vi "Omniax_mDrive_COM9_MM_BR_RES.vi"() -> ()   [LabVIEW 2009]
uses:
  <vilib>/Instr/_visa.llb/VISA Configure Serial Port (Instr).vi
panel:
  out "Y Backlash corr":bool
  in  "Y Scan set":bool
  in  "Y Scan Velocity SP mm/sec":dbl
  in  "Y Scan Length SP mm":dbl
  in  "Y Move Set":bool
  out "Y Backlash steps/sec":i32
  out "Y Backlash":i32
  out "Y in Motion":bool
  in  "Reset":bool
  out "Reset Y Motor Steps":i32
  in  "Reset Y Position mm":dbl
  out "Y Velocity MV mm/sec":dbl
  in  "Y Velocity SP mm/sec":dbl
  in  "Y Position SP mm":dbl
  out "Y Position MV mm":dbl
  out "Y Holding Current %":i32
  out "Y Run Current %":i32
  out "Y Scan velocity MV mm/sec":dbl format="%#_6f"
  out "Y Scan length MV mm":dbl
  in  "Y Scan Cancel":bool
  out "Y Position mm PV":dbl
  out "Y offset mm":dbl
  out "Y mm/rev":dbl
  out "Y steps/rev":u32
  out "Y scan steps/sec MV step/sec":i32
  in  "Y Scan Length SP steps":i32 min=-460800 max=460800 step=100
  out "Y Scan":bool
  in  "Y Scan Set":bool
  in  "Scan Go":bool
  in  "Y Velocity SP step/sec":i32 min=1 max=102400
  in  "Y Scan Velocity SP steps/sec":i32=1 min=1 max=102400 step=1
  in  "Stop":bool
  out "Y in Range":bool
  out "Y Step PV":i32 max=2000
  in  "Go":bool
  in  "Y Step SP":i32=-20000 min=-460800 max=460800 step=500
  out "Y MINPOS":i32=-94296
  out "Y MAXPOS":i32=-34296
  out "Y COM PORT":refnum<visa-resource-name>="COM5"
  # "MY"
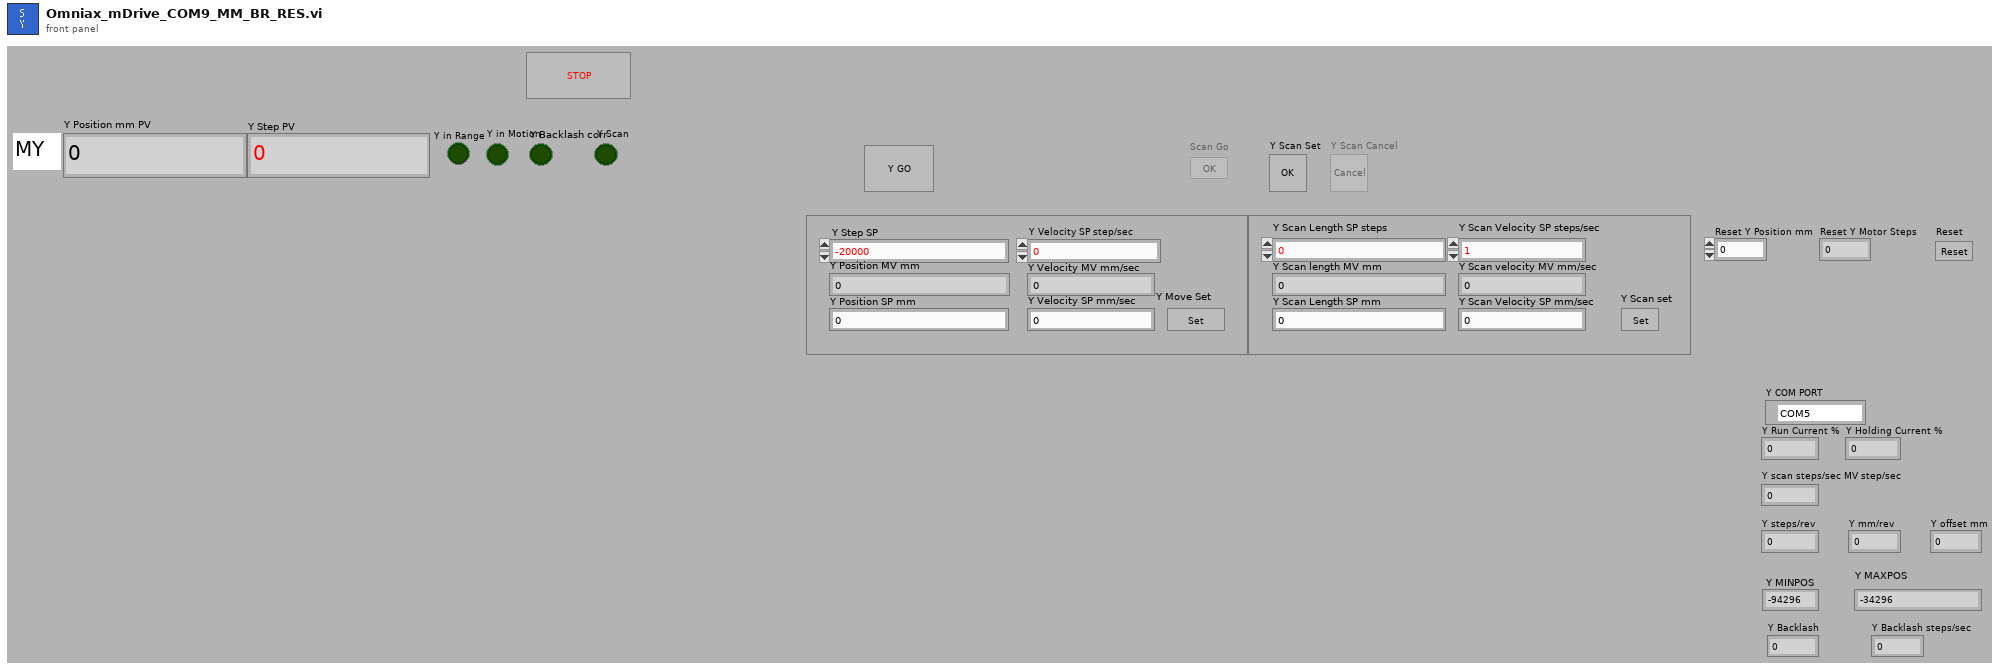
[diagram p1: front panel]
types:
  T1 = enum8{"Enabled", "Disabled", "Disabled and Grayed Out"}
  T2 = enum16{"Stop", "Reset", "Run Current", "Holding Current", "Accel Rate", "Decel Rate", "Move to Relative Position", "Move to Absolute Position", "Echo Mode", "Print Parameter", "Send String", "Microstep Resolution", "Set Current Position", "Max Velocity"}
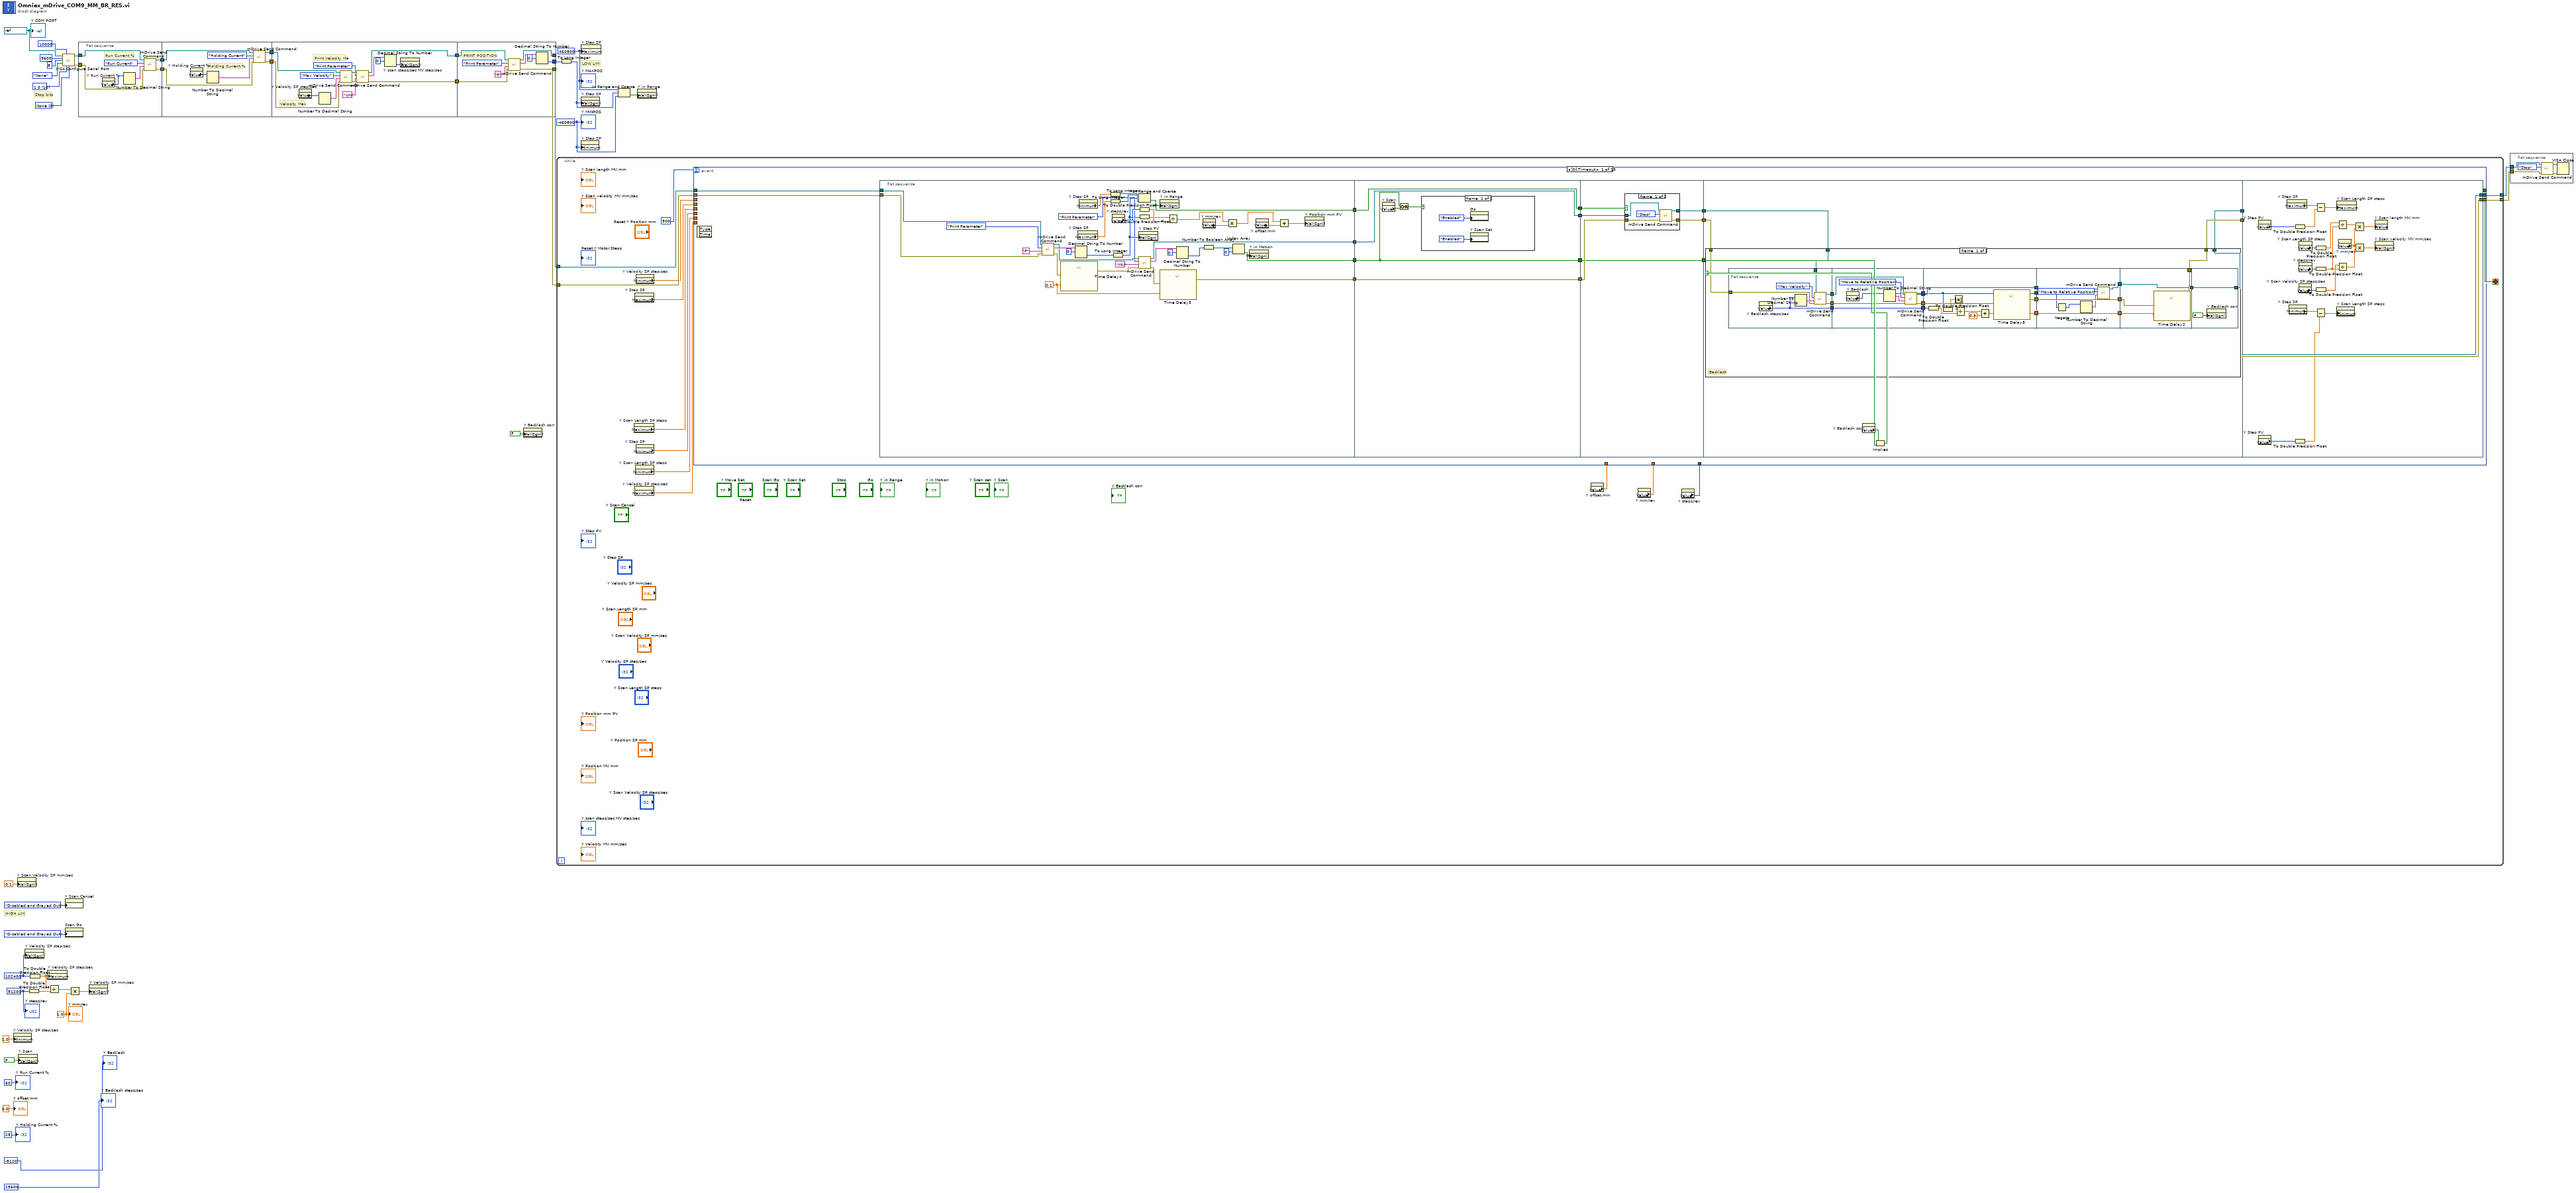
[diagram p0: block diagram]
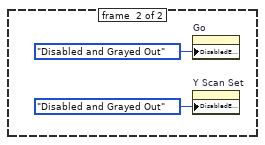
[diagram p2: hidden frame]
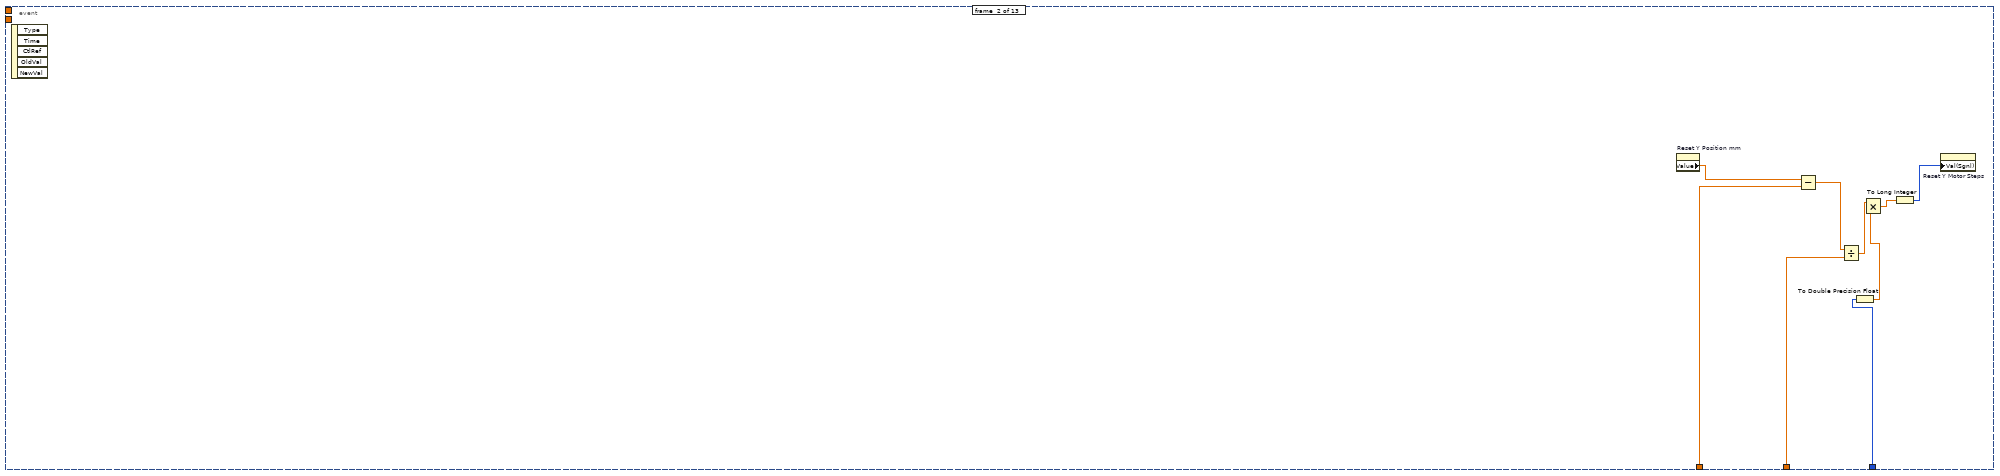
[diagram p5: hidden frame]
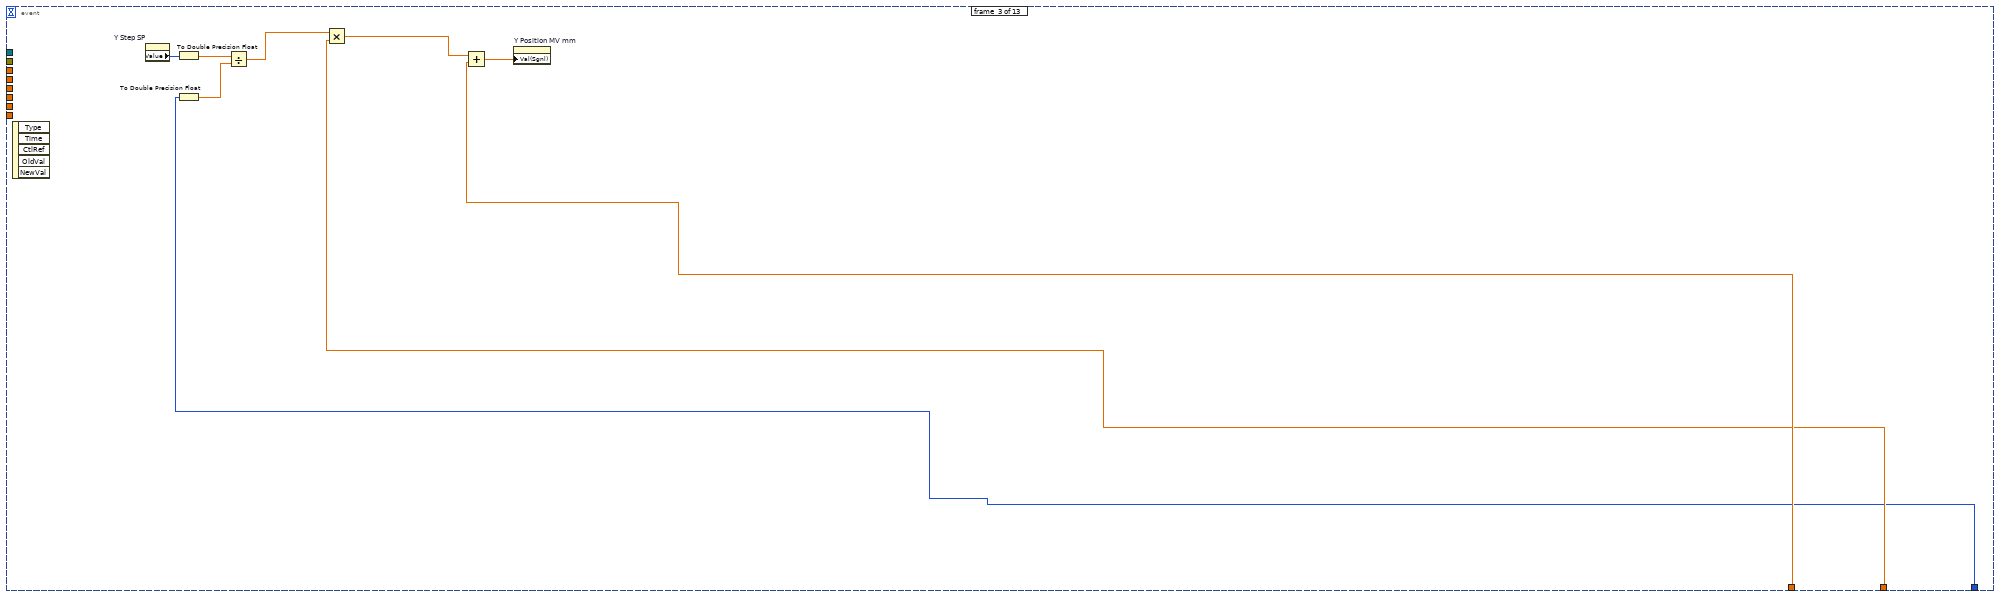
[diagram p6: hidden frame]
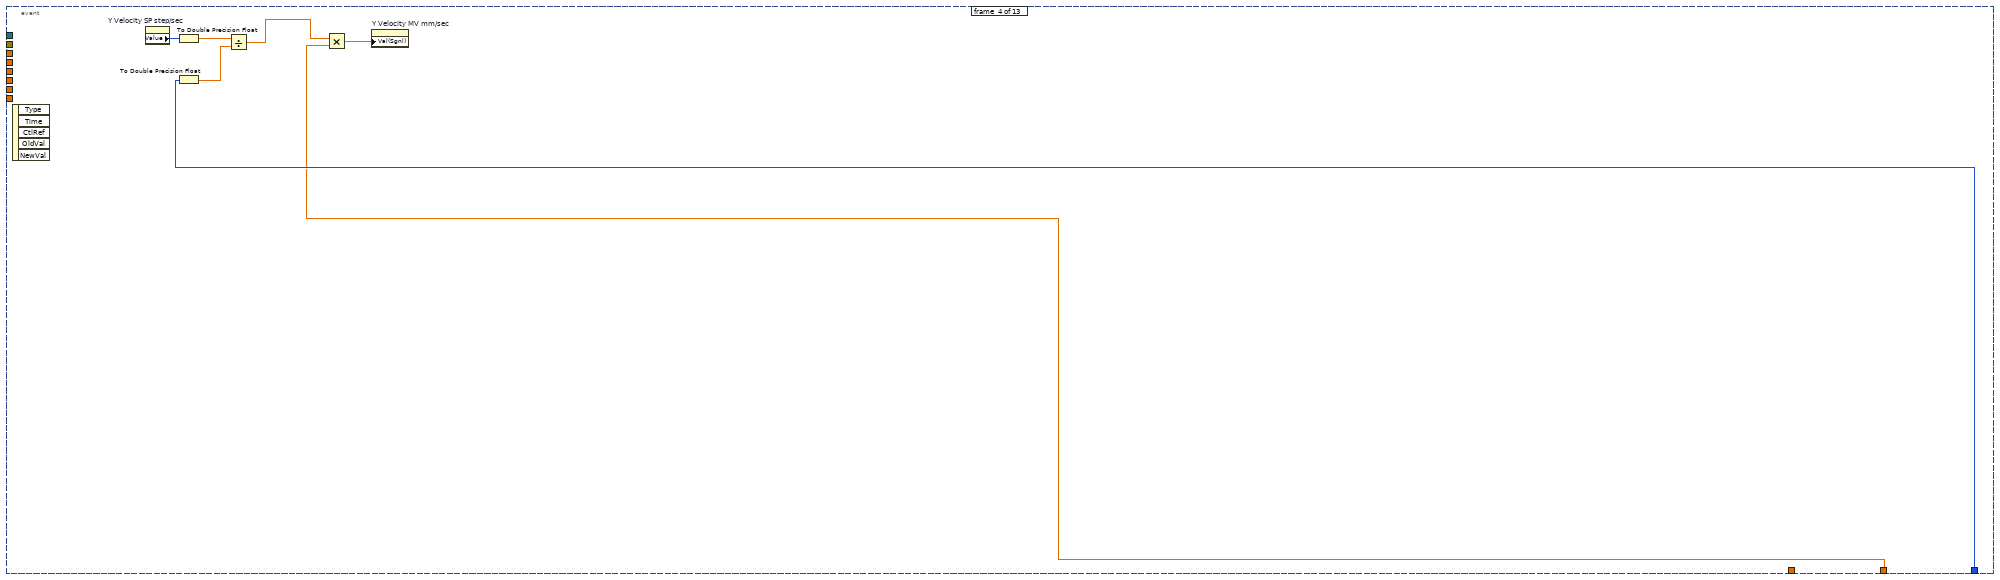
[diagram p7: hidden frame]
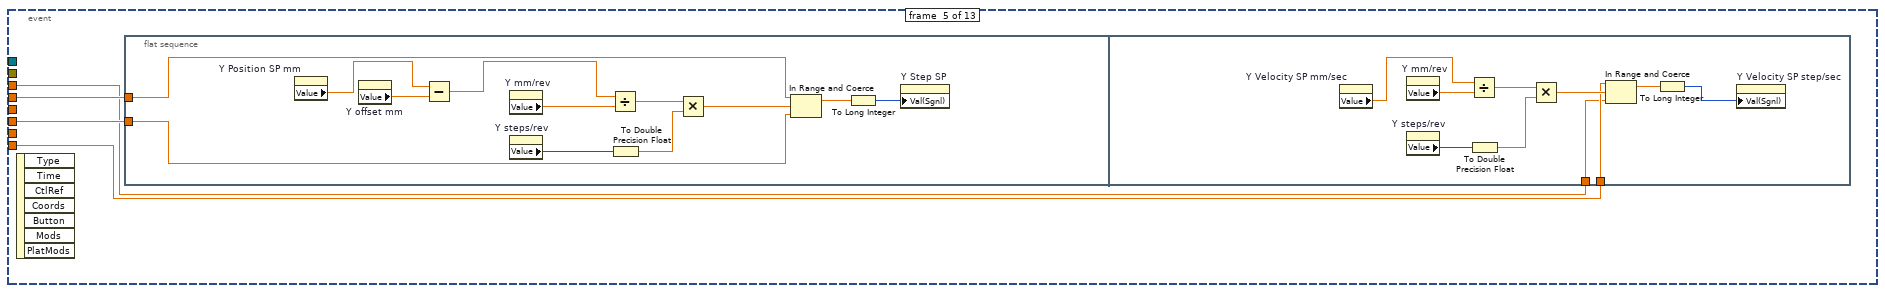
[diagram p8: hidden frame]
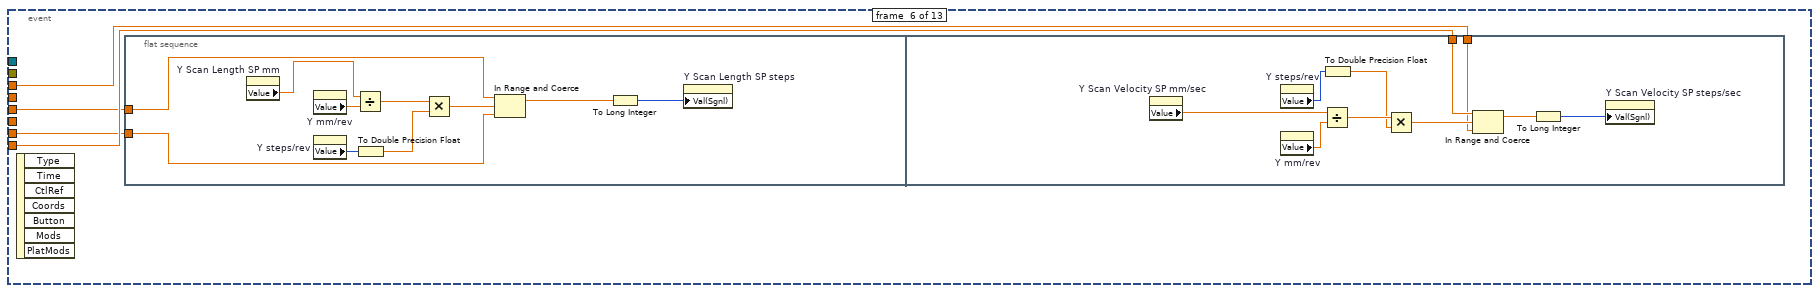
[diagram p9: hidden frame]
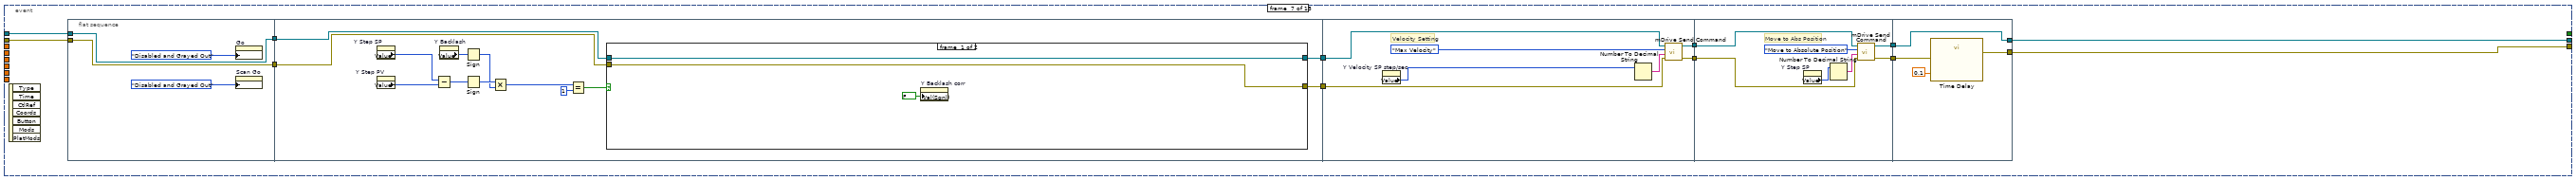
[diagram p10: hidden frame]
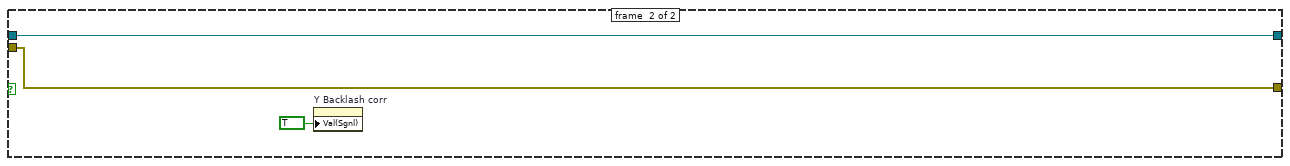
[diagram p11: hidden frame]
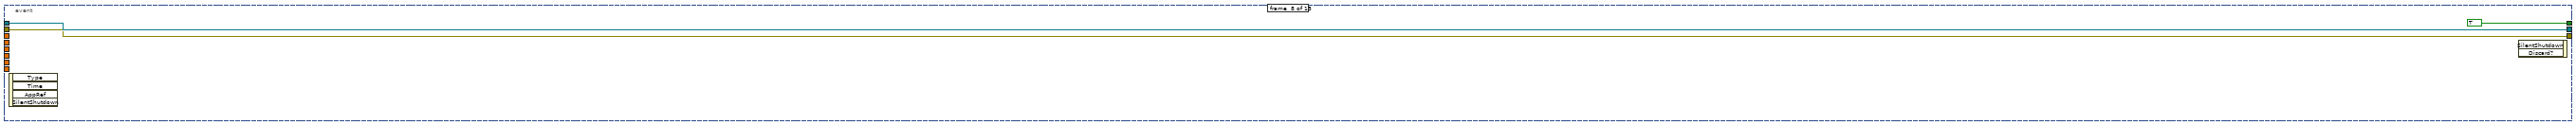
[diagram p12: hidden frame]
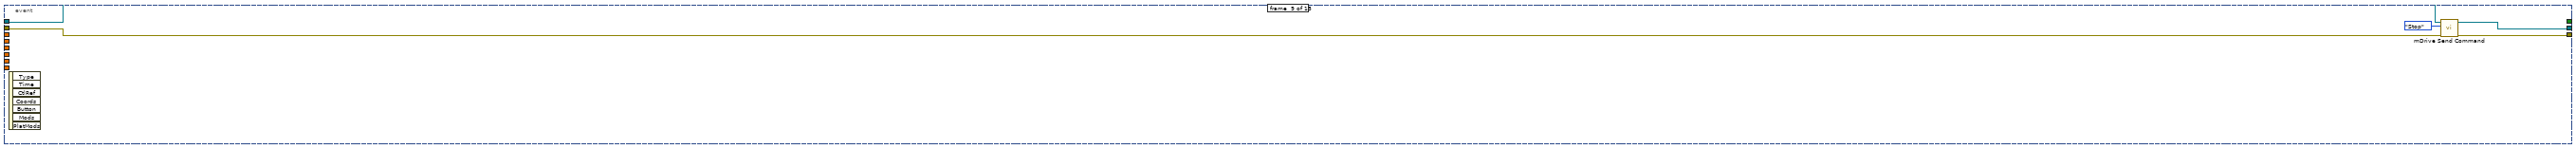
[diagram p13: hidden frame]
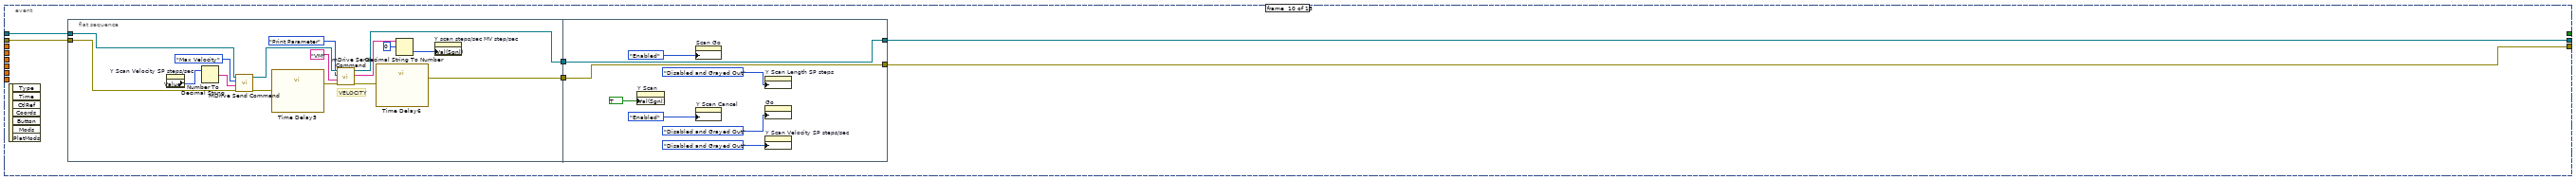
[diagram p14: hidden frame]
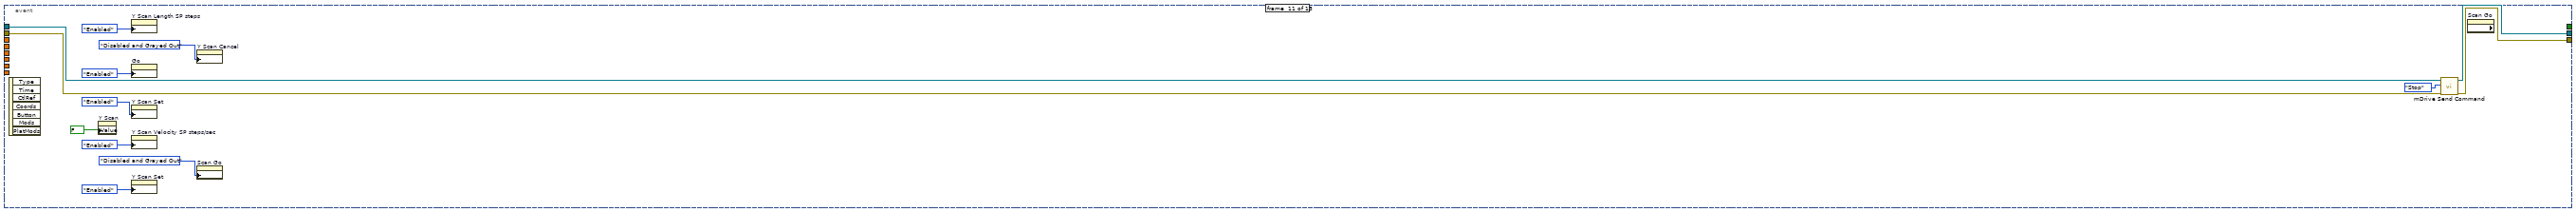
[diagram p15: hidden frame]
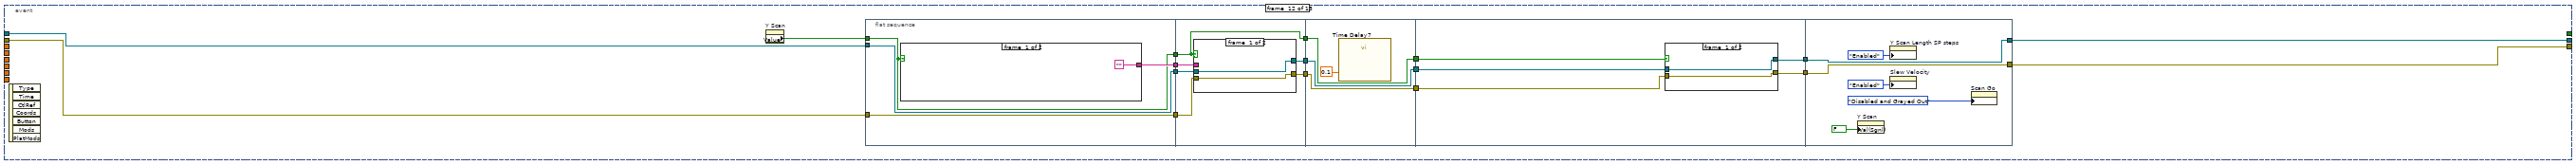
[diagram p16: hidden frame]
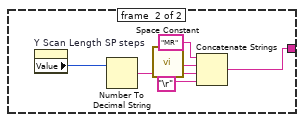
[diagram p17: hidden frame]
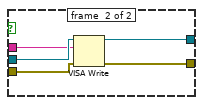
[diagram p18: hidden frame]
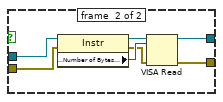
[diagram p19: hidden frame]
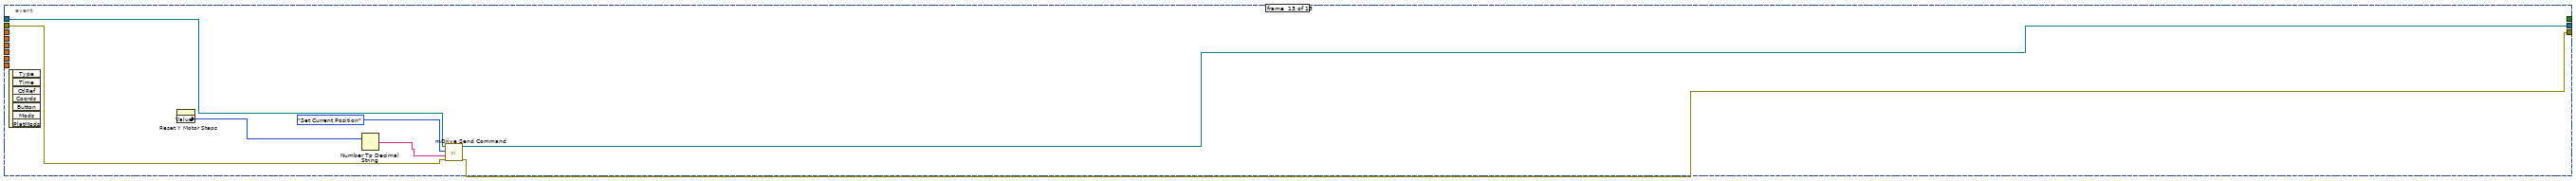
[diagram p20: hidden frame]
diagram:
  w9 = 1.0 ("MM/rev")
  w6 = u32 51200 ("step/rev")
  w11 = 102400 ("Value (Signaling)")
  w29 = -460800 ("lower limit")
  w28 = 460800 ("upper limit")
  w36 = refnum<visa-resource-name> "COM9" ("COM PORT")
  w38 = u16 0 items=["None", "XON/XOFF", "RTS/CTS", "XON/XOFF & RTS/CTS", "DTR/DSR", "XON/XOFF & DTR/DSR"] ("flow control (0:none)")
  w39 = u16 10 items=["1.0"=10, "1.5"=15, "2.0"=20] ("stop bits (10: 1 bit)")
  # "HIGH LIM"
  # "LOW LIM"
  # "Stop bits"
  n1 = property on="Y Velocity SP step/sec" class="DigNum (strict)"("Minimum"=1.0 ("Data Entry Limits:Minimum")) -> ()  [unwired: 2 in, 2 out]
  n2 = property on="Y Scan Velocity SP mm/sec" class="DigNum (strict)"("Val(Sgnl)"=0.1 ("Value (Signaling)")) -> ()  [unwired: 2 in, 2 out]
  n3 = property on="Y Scan" class="Bool (strict)"("Val(Sgnl)"=FALSE ("Value (Signaling)")) -> ()  [unwired: 2 in, 2 out]
  n4 = property on="Y Velocity SP step/sec" class="DigNum (strict)"("Val(Sgnl)"=w11) -> ()  [unwired: 2 in, 2 out]
  n5 = To Double Precision Float(number=w6) -> (double precision float=w7:dbl)
  n6 = To Double Precision Float(number=w11) -> (double precision float=w5:dbl)
  n7 = property on="Y Velocity SP step/sec" class="DigNum (strict)"("Maximum"=w5) -> ()  [unwired: 2 in, 2 out]
  n8 = Divide(x=w5, y=w7) -> (x/y=w10:dbl)
  n9 = call-poly "VISA Configure Serial Port"("VISA resource name"=w36, "timeout (10sec)"=u32 10000, "baud rate (9600)"=u32 9600, "data bits (8)"=u16 8, "parity (0:none)"=enum16{"None", "Odd", "Even", "Mark", "Space"}."None", "stop bits (10: 1 bit)"=w39, "flow control (0:none)"=w38) -> ("VISA resource name out"=w24:refnum<visa-resource-name>, "error out"=w23:errorcluster)  [unwired: 7 in]
  n10 = property on="Y Scan Cancel" class="Bool"("DisabledEnum"=T1."Disabled and Grayed Out" ("Disabled")) -> ()  [unwired: 2 in, 2 out]
  n11 = property on="Scan Go" class="Bool"("DisabledEnum"=T1."Disabled and Grayed Out" ("Disabled")) -> ()  [unwired: 2 in, 2 out]
  n12 = Multiply(x=w10, y=w9) -> (x*y=w8:dbl)
  n13 = flat-sequence {
    tunnel: w23 -> [w49]
    tunnel: w24 -> [w47]
    tunnel: [w46] -> w18
    tunnel: [w48] -> w16
    tunnel: w18 -> [w56]
    tunnel: [w55] -> w17
    tunnel: w16 -> [w53]
    tunnel: [w54] -> w15
    tunnel: [w66] -> w26
    tunnel: [w67] -> w25
    tunnel: w17 -> [w65]
    tunnel: w15 -> [w64]
    tunnel: [w79] -> w35
    tunnel: [w78] -> w34
    tunnel: [w73] -> w27
    tunnel: w26 -> [w77]
    tunnel: w25 -> [w76]
    frame #0 {
      # "Run Current %"
      n14 = property on="Y Run Current %" class="DigNum (strict)"() -> ("Value"=w44:i32)  [unwired: 2 in, 2 out]
      n15 = Number To Decimal String(number=w44) -> (decimal integer string=w45:string)  [unwired: 1 in]
      n16 = call "mDrive Send Command.vi"("error in (no error)"=w49, "Extra"=w45, "Command"=T2."Run Current", "VISA resource name"=w47) -> ("error out"=w48:errorcluster, "VISA resource name out"=w46:refnum<visa-resource-name>)  [unwired: 3 in, 1 out]
    }
    frame #1 {
      # "Holding Current %"
      n17 = property on="Y Holding Current %" class="DigNum (strict)"() -> ("Value"=w51:i32)  [unwired: 2 in, 2 out]
      n18 = Number To Decimal String(number=w51) -> (decimal integer string=w52:string)  [unwired: 1 in]
      n19 = call "mDrive Send Command.vi"("error in (no error)"=w53, "Extra"=w52, "Command"=T2."Holding Current", "VISA resource name"=w56) -> ("error out"=w54:errorcluster, "VISA resource name out"=w55:refnum<visa-resource-name>)  [unwired: 3 in, 1 out]
    }
    frame #2 {
      # "Print Velocity Ma"
      # "Velocity Max"
      n20 = property on="Y Velocity SP step/sec" class="DigNum (strict)"() -> ("Value"=w63:i32)  [unwired: 2 in, 2 out]
      n21 = Number To Decimal String(number=w63) -> (decimal integer string=w62:string)  [unwired: 1 in]
      n22 = call "mDrive Send Command.vi"("error in (no error)"=w64, "Extra"=w62, "Command"=T2."Max Velocity", "VISA resource name"=w65) -> ("error out"=w60:errorcluster, "VISA resource name out"=w70:refnum<visa-resource-name>)  [unwired: 3 in, 1 out]
      n23 = call "mDrive Send Command.vi"("error in (no error)"=w60, "Extra"="VM", "Command"=T2."Print Parameter", "VISA resource name"=w70) -> ("error out"=w67:errorcluster, "read buffer"=w68:string, "VISA resource name out"=w66:refnum<visa-resource-name>)  [unwired: 3 in]
      n24 = Decimal String To Number(string=w68, offset=0) -> (number=w61:i32)  [unwired: 1 in, 1 out]
      n25 = property on="Y scan steps/sec MV step/sec" class="DigNum (strict)"("Val(Sgnl)"=w61) -> ()  [unwired: 2 in, 2 out]
    }
    frame #3 {
      # "PRINT POSITION"
      n26 = call "mDrive Send Command.vi"("error in (no error)"=w76, "Extra"="P", "Command"=T2."Print Parameter", "VISA resource name"=w77) -> ("error out"=w78:errorcluster, "read buffer"=w75:string, "VISA resource name out"=w79:refnum<visa-resource-name>)  [unwired: 3 in]
      n27 = Decimal String To Number(string=w75, offset=0) -> (number=w73:i32)  [unwired: 1 in, 1 out]
    }
  }
  n28 = property on="Y Velocity SP mm/sec" class="DigNum (strict)"("Val(Sgnl)"=w8) -> ()  [unwired: 2 in, 2 out]
  n29 = property on="Y Backlash corr" class="Bool (strict)"("Val(Sgnl)"=FALSE ("Value (Signaling)")) -> ()  [unwired: 2 in, 2 out]
  n30 = while {
    tunnel: w35 -> [w90]
    tunnel: w34 -> [w93]
    tunnel: [w94] -> w31
    tunnel: [w92] -> w32
    stop <- w89 stop-if-true
    n31 = property on="Y Scan Length SP steps" class="DigNum (strict)"() -> ("Maximum"=w83:dbl)  [unwired: 2 in, 2 out]
    n32 = property on="Y Step SP" class="DigNum (strict)"() -> ("Maximum"=w87:dbl)  [unwired: 2 in, 2 out]
    n33 = property on="Y Velocity SP step/sec" class="DigNum (strict)"() -> ("Maximum"=w86:dbl)  [unwired: 2 in, 2 out]
    n34 = property on="Y Scan Length SP steps" class="DigNum (strict)"() -> ("Minimum"=w84:dbl)  [unwired: 2 in, 2 out]
    n35 = property on="Y Velocity SP step/sec" class="DigNum (strict)"() -> ("Minimum"=w85:dbl)  [unwired: 2 in, 2 out]
    n36 = property on="Y Step SP" class="DigNum (strict)"() -> ("Minimum"=w88:dbl)  [unwired: 2 in, 2 out]
    n37 = property on="Y offset mm" class="DigNum (strict)"() -> ("Value"=w82:dbl)  [unwired: 2 in, 2 out]
    n38 = property on="Y mm/rev" class="DigNum (strict)"() -> ("Value"=w81:dbl)  [unwired: 2 in, 2 out]
    n39 = property on="Y steps/rev" class="DigNum (strict)"() -> ("Value"=w80:u32)  [unwired: 2 in, 2 out]
    n40 = event shown="[0] Timeout" {
      selector: _ -> [_ _ _ _ _ _ _ _ _ _ _ _ _]
      dyn-events: _ -> [_ _ _ _ _ _ _ _ _ _ _ _ _]
      timeout: 500 -> [_ _ _ _ _ _ _ _ _ _ _ _ _]
      tunnel: w93 -> [w111 _ _ _ _ _ w339 w389 w394 w401 w431 w455 w506]
      tunnel: [w110 _ _ _ _ _ w345 w389 w392 w399 w433 w452 w504] -> w94
      tunnel: w90 -> [w108 _ _ _ _ _ w340 w390 w395 w400 w432 w454 w507]
      tunnel: [w109 _ _ _ _ _ w346 w390 w393 w396 w434 w453 w505] -> w92
      tunnel: [_ _ _ _ _ _ _ TRUE _ _ _ _ _] -> w89
      tunnel: w88 -> [_ _ _ _ w288 _ _ _ _ _ _ _ _]
      tunnel: w87 -> [_ _ _ _ w287 _ _ _ _ _ _ _ _]
      tunnel: w86 -> [_ _ _ _ w286 w314 _ _ _ _ _ _ _]
      tunnel: w85 -> [_ _ _ _ w285 w313 _ _ _ _ _ _ _]
      tunnel: w84 -> [_ _ _ _ _ w312 _ _ _ _ _ _ _]
      tunnel: w83 -> [_ _ _ _ _ w311 _ _ _ _ _ _ _]
      tunnel: w82 -> [_ w267 w271 _ _ _ _ _ _ _ _ _ _]
      tunnel: w81 -> [_ w265 w270 w278 _ _ _ _ _ _ _ _ _]
      tunnel: w80 -> [_ w263 w269 w279 _ _ _ _ _ _ _ _ _]
      event #0 {
        n41 = event-data() -> ()  [unwired: 1 in, 2 out]
        n42 = flat-sequence {
          tunnel: w111 -> [w142]
          tunnel: w108 -> [w141]
          tunnel: [w147] -> w107
          tunnel: [w121] -> w105
          tunnel: [w134] -> w103
          tunnel: [w112] -> w101
          tunnel: w107 -> [w153]
          tunnel: [w153] -> w106
          tunnel: w105 -> [w152]
          tunnel: [w152] -> w104
          tunnel: w103 -> [w151]
          tunnel: [w151] -> w102
          tunnel: w101 -> [w148]
          tunnel: [w148] -> w96
          tunnel: w106 -> [w160]
          tunnel: [w161] -> w100
          tunnel: w104 -> [w163]
          tunnel: [w162] -> w99
          tunnel: w102 -> [w159]
          tunnel: [w158] -> w97
          tunnel: w96 -> [w158]
          tunnel: w100 -> [w173]
          tunnel: w99 -> [w174]
          tunnel: [w172] -> w98
          tunnel: w97 -> [w176]
          tunnel: [w171] -> w95
          tunnel: [w258] -> w110
          tunnel: [w259] -> w109
          tunnel: w98 -> [w258]
          tunnel: w95 -> [w259]
          frame #0 {
            w116 = 0.1 ("Delay Time (s)")
            n43 = call "mDrive Send Command.vi"("error in (no error)"=w142, "Extra"="P", "Command"=T2."Print Parameter", "VISA resource name"=w141) -> ("error out"=w140:errorcluster, "read buffer"=w146:string, "VISA resource name out"=w144:refnum<visa-resource-name>)  [unwired: 3 in]
            n44 = call "Time Delay4"("error in (no error)"=w140, "Delay Time (s)"=w116) -> ("error out"=w139:errorcluster)  [unwired: 9 in]
            n45 = Decimal String To Number(string=w146, offset=0) -> (number=w124:i32)  [unwired: 1 in, 1 out]
            n46 = property on="Y Step SP" class="DigNum (strict)"() -> ("Maximum"=w136:dbl)  [unwired: 2 in, 2 out]
            n47 = property on="Y Step SP" class="DigNum (strict)"() -> ("Minimum"=w138:dbl)  [unwired: 2 in, 2 out]
            n48 = To Long Integer(number=w138) -> (32bit integer=w137:i32)
            n49 = To Long Integer(number=w136) -> (32bit integer=w135:i32)
            n50 = To Long Integer(number=w124) -> (32bit integer=w126:i32)
            n51 = property on="Y steps/rev" class="DigNum (strict)"() -> ("Value"=w132:u32)  [unwired: 2 in, 2 out]
            n52 = In Range and Coerce(upper limit=w135, x=w126, lower limit=w137) -> (In Range?=w134:bool)  [unwired: 1 out]
            n53 = To Double Precision Float(number=w132) -> (double precision float=w133:dbl)
            n54 = To Double Precision Float(number=w126) -> (double precision float=w127:dbl)
            n55 = property on="Y Step PV" class="DigNum (strict)"("Val(Sgnl)"=w126) -> ()  [unwired: 2 in, 2 out]
            n56 = call "mDrive Send Command.vi"("error in (no error)"=w139, "Extra"="MV", "Command"=T2."Print Parameter", "VISA resource name"=w144) -> ("error out"=w143:errorcluster, "read buffer"=w122:string, "VISA resource name out"=w147:refnum<visa-resource-name>)  [unwired: 3 in]
            n57 = property on="Y in Range" class="Bool (strict)"("Val(Sgnl)"=w134) -> ()  [unwired: 2 in, 2 out]
            n58 = call "Time Delay3"("error in (no error)"=w143, "Delay Time (s)"=w116) -> ("error out"=w121:errorcluster)  [unwired: 9 in]
            n59 = Divide(x=w127, y=w133) -> (x/y=w131:dbl)
            n60 = Decimal String To Number(string=w122, offset=0 ("offset (0)")) -> (number=w115:i32)  [unwired: 1 in, 1 out]
            n61 = property on="Y mm/rev" class="DigNum (strict)"() -> ("Value"=w130:dbl)  [unwired: 2 in, 2 out]
            n62 = Number To Boolean Array(number=w115) -> (Boolean array=w114:bool[])
            n63 = Multiply(x=w131, y=w130) -> (x*y=w129:dbl)
            n64 = Index Array(array=w114, index=0) -> (element=w112:bool)
            n65 = property on="Y in Motion" class="Bool (strict)"("Val(Sgnl)"=w112) -> ()  [unwired: 2 in, 2 out]
            n66 = property on="Y offset mm" class="DigNum (strict)"() -> ("Value"=w128:dbl)  [unwired: 2 in, 2 out]
            n67 = Add(x=w129, y=w128) -> (x+y=w125:dbl)
            n68 = property on="Y Position mm PV" class="DigNum (strict)"("Val(Sgnl)"=w125) -> ()  [unwired: 2 in, 2 out]
          }
          frame #1 {
            n69 = property on="Y Scan" class="Bool (strict)"() -> ("Value"=w149:bool)  [unwired: 2 in, 2 out]
            n70 = Or(x=w148, y=w149) -> (x .or. y?=w150:bool)
            n71 = case shown="False" w150 {
              frame #0 {
                n72 = property on="Go" class="Bool"("DisabledEnum"=T1."Enabled" ("Disabled")) -> ()  [unwired: 2 in, 2 out]
                n73 = property on="Y Scan Set" class="Bool"("DisabledEnum"=T1."Enabled" ("Disabled")) -> ()  [unwired: 2 in, 2 out]
              }
              frame #1 {
                n74 = property on="Go" class="Bool"("DisabledEnum"=T1."Disabled and Grayed Out" ("Disabled")) -> ()  [unwired: 2 in, 2 out]
                n75 = property on="Y Scan Set" class="Bool"("DisabledEnum"=T1."Disabled and Grayed Out" ("Disabled")) -> ()  [unwired: 2 in, 2 out]
              }
            }
          }
          frame #2 {
            n76 = case shown="False" w159 {
              tunnel: w160 -> [w166 w170]
              tunnel: [w167 w170] -> w161
              tunnel: [w168 w169] -> w162
              tunnel: w163 -> [w165 w169]
              frame #0 {
                n77 = call "mDrive Send Command.vi"("error in (no error)"=w165, "Command"=T2."Stop", "VISA resource name"=w166) -> ("error out"=w168:errorcluster, "VISA resource name out"=w167:refnum<visa-resource-name>)  [unwired: 4 in, 1 out]
              }
              frame #1 {
              }
            }
          }
          frame #3 {
            n78 = property on="Y Backlash corr" class="Bool (strict)"() -> ("Value"=w177:bool)  [unwired: 2 in, 2 out]
            n79 = Implies(1:w176, 2:w177) -> (0:w175:bool)
            n80 = case shown="False" w175 {
              tunnel: w174 -> [w184 w237]
              tunnel: w173 -> [w183 w238]
              tunnel: [w182 w237] -> w172
              tunnel: [w181 w238] -> w171
              frame #0 {
                # "Backlash"
                n81 = flat-sequence {
                  tunnel: [w199] -> w196
                  tunnel: [w201] -> w195
                  tunnel: [w200] -> w194
                  tunnel: w184 -> [w198]
                  tunnel: w183 -> [w197]
                  tunnel: w196 -> [w209]
                  tunnel: [w209] -> w193
                  tunnel: w195 -> [w208]
                  tunnel: w194 -> [w207]
                  tunnel: [w206] -> w192
                  tunnel: [w205] -> w191
                  tunnel: [w204] -> w180
                  tunnel: w193 -> [w219]
                  tunnel: w192 -> [w218]
                  tunnel: w191 -> [w216]
                  tunnel: [w217] -> w190
                  tunnel: [w216] -> w189
                  tunnel: [w215] -> w186
                  tunnel: [w214] -> w185
                  tunnel: w180 -> [w214]
                  tunnel: w190 -> [w230]
                  tunnel: w189 -> [w223]
                  tunnel: [w230] -> w188
                  tunnel: [w229] -> w187
                  tunnel: w186 -> [w229]
                  tunnel: w185 -> [w225]
                  tunnel: [w224] -> w178
                  tunnel: w188 -> [w234]
                  tunnel: w187 -> [w233]
                  tunnel: [w232] -> w182
                  tunnel: [w231] -> w179
                  tunnel: w178 -> [w231]
                  tunnel: [w236] -> w181
                  tunnel: w179 -> [w236]
                  frame #0 {
                    n82 = property on="Y Backlash steps/sec" class="DigNum (strict)"() -> ("Value"=w199:i32)  [unwired: 2 in, 2 out]
                    n83 = Number To Decimal String(number=w199) -> (decimal integer string=w202:string)  [unwired: 1 in]
                    n84 = call "mDrive Send Command.vi"("error in (no error)"=w198, "Extra"=w202, "Command"=T2."Max Velocity", "VISA resource name"=w197) -> ("error out"=w200:errorcluster, "VISA resource name out"=w201:refnum<visa-resource-name>)  [unwired: 3 in, 1 out]
                  }
                  frame #1 {
                    n85 = property on="Y Backlash" class="DigNum (strict)"() -> ("Value"=w204:i32)  [unwired: 2 in, 2 out]
                    n86 = Number To Decimal String(number=w204) -> (decimal integer string=w210:string)  [unwired: 1 in]
                    n87 = call "mDrive Send Command.vi"("error in (no error)"=w207, "Extra"=w210, "Command"=T2."Move to Relative Position", "VISA resource name"=w208) -> ("error out"=w206:errorcluster, "VISA resource name out"=w205:refnum<visa-resource-name>)  [unwired: 3 in, 1 out]
                  }
                  frame #2 {
                    n88 = To Double Precision Float(number=w219) -> (double precision float=w221:dbl)
                    n89 = To Double Precision Float(number=w214) -> (double precision float=w212:dbl)
                    n90 = Absolute Value(x=w212) -> (abs(x)=w213:dbl)
                    n91 = Divide(x=w213, y=w221) -> (x/y=w222:dbl)
                    n92 = Add(x=w222, y=0.3) -> (x+y=w215:dbl)
                    n93 = call "Time Delay8"("error in (no error)"=w218, "Delay Time (s)"=w215) -> ("error out"=w217:errorcluster)  [unwired: 9 in]
                  }
                  frame #3 {
                    n94 = Negate(x=w225) -> (-x=w226:i32)
                    n95 = Number To Decimal String(number=w226) -> (decimal integer string=w227:string)  [unwired: 1 in]
                    n96 = call "mDrive Send Command.vi"("Extra"=w227, "Command"=T2."Move to Relative Position", "VISA resource name"=w223) -> ("VISA resource name out"=w224:refnum<visa-resource-name>)  [unwired: 4 in, 2 out]
                  }
                  frame #4 {
                    n97 = call "Time Delay2"("error in (no error)"=w234, "Delay Time (s)"=w233) -> ("error out"=w232:errorcluster)  [unwired: 9 in]
                  }
                  frame #5 {
                    n98 = property on="Y Backlash corr" class="Bool (strict)"("Val(Sgnl)"=FALSE ("Value (Signaling)")) -> ()  [unwired: 2 in, 2 out]
                  }
                }
              }
              frame #1 {
              }
            }
          }
          frame #4 {
            n99 = property on="Y Step PV" class="DigNum (strict)"() -> ("Value"=w248:i32)  [unwired: 2 in, 2 out]
            n100 = property on="Y Step PV" class="DigNum (strict)"() -> ("Value"=w246:i32)  [unwired: 2 in, 2 out]
            n101 = property on="Y Step SP" class="DigNum (strict)"() -> ("Maximum"=w255:dbl)  [unwired: 2 in, 2 out]
            n102 = property on="Y Step SP" class="DigNum (strict)"() -> ("Minimum"=w256:dbl)  [unwired: 2 in, 2 out]
            n103 = To Double Precision Float(number=w248) -> (double precision float=w247:dbl)
            n104 = To Double Precision Float(number=w246) -> (double precision float=w245:dbl)
            n105 = property on="Y Scan Velocity SP steps/sec" class="DigNum (strict)"() -> ("Value"=w243:i32)  [unwired: 2 in, 2 out]
            n106 = property on="Y Scan Length SP steps" class="DigNum (strict)"() -> ("Value"=w252:i32)  [unwired: 2 in, 2 out]
            n107 = property on="Y steps/rev" class="DigNum (strict)"() -> ("Value"=w250:u32)  [unwired: 2 in, 2 out]
            n108 = Subtract(x=w255, y=w247) -> (x-y=w254:dbl)
            n109 = Subtract(x=w256, y=w245) -> (x-y=w257:dbl)
            n110 = To Double Precision Float(number=w252) -> (double precision float=w251:dbl)
            n111 = To Double Precision Float(number=w250) -> (double precision float=w244:dbl)
            n112 = To Double Precision Float(number=w243) -> (double precision float=w242:dbl)
            n113 = property on="Y Scan Length SP steps" class="DigNum (strict)"("Maximum"=w254) -> ()  [unwired: 2 in, 2 out]
            n114 = Divide(x=w251, y=w244) -> (x/y=w253:dbl)
            n115 = Divide(x=w242, y=w244) -> (x/y=w241:dbl)
            n116 = property on="Y Scan Length SP steps" class="DigNum (strict)"("Minimum"=w257) -> ()  [unwired: 2 in, 2 out]
            n117 = property on="Y mm/rev" class="DigNum (strict)"() -> ("Value"=w249:dbl)  [unwired: 2 in, 2 out]
            n118 = Multiply(x=w253, y=w249) -> (x*y=w240:dbl)
            n119 = Multiply(x=w249, y=w241) -> (x*y=w239:dbl)
            n120 = property on="Y Scan length MV mm" class="DigNum (strict)"("Value"=w240) -> ()  [unwired: 2 in, 2 out]
            n121 = property on="Y Scan velocity MV mm/sec" class="DigNum (strict)"("Val(Sgnl)"=w239) -> ()  [unwired: 2 in, 2 out]
          }
        }
      }
      event #1 {
        n122 = event-data() -> ()  [unwired: 1 in, 5 out]
        n123 = property on="Reset Y Position mm" class="DigNum (strict)"() -> ("Value"=w268:dbl)  [unwired: 2 in, 2 out]
        n124 = Subtract(x=w268, y=w267) -> (x-y=w266:dbl)
        n125 = Divide(x=w266, y=w265) -> (x/y=w264:dbl)
        n126 = To Double Precision Float(number=w263) -> (double precision float=w262:dbl)
        n127 = Multiply(x=w264, y=w262) -> (x*y=w261:dbl)
        n128 = To Long Integer(number=w261) -> (32bit integer=w260:i32)
        n129 = property on="Reset Y Motor Steps" class="DigNum (strict)"("Val(Sgnl)"=w260) -> ()  [unwired: 2 in, 2 out]
      }
      event #2 {
        n130 = event-data() -> ()  [unwired: 1 in, 5 out]
        n131 = property on="Y Step SP" class="DigNum (strict)"() -> ("Value"=w273:i32)  [unwired: 2 in, 2 out]
        n132 = To Double Precision Float(number=w273) -> (double precision float=w274:dbl)
        n133 = To Double Precision Float(number=w269) -> (double precision float=w277:dbl)
        n134 = Divide(x=w274, y=w277) -> (x/y=w276:dbl)
        n135 = Multiply(x=w276, y=w270) -> (x*y=w275:dbl)
        n136 = Add(x=w275, y=w271) -> (x+y=w272:dbl)
        n137 = property on="Y Position MV mm" class="DigNum (strict)"("Val(Sgnl)"=w272) -> ()  [unwired: 2 in, 2 out]
      }
      event #3 {
        n138 = event-data() -> ()  [unwired: 1 in, 5 out]
        n139 = property on="Y Velocity SP step/sec" class="DigNum (strict)"() -> ("Value"=w281:i32)  [unwired: 2 in, 2 out]
        n140 = To Double Precision Float(number=w281) -> (double precision float=w282:dbl)
        n141 = To Double Precision Float(number=w279) -> (double precision float=w284:dbl)
        n142 = Divide(x=w282, y=w284) -> (x/y=w283:dbl)
        n143 = Multiply(x=w283, y=w278) -> (x*y=w280:dbl)
        n144 = property on="Y Velocity MV mm/sec" class="DigNum (strict)"("Val(Sgnl)"=w280) -> ()  [unwired: 2 in, 2 out]
      }
      event #4 {
        n145 = event-data() -> ()  [unwired: 1 in, 7 out]
        n146 = flat-sequence {
          tunnel: w288 -> [w291]
          tunnel: w287 -> [w290]
          tunnel: w286 -> [w303]
          tunnel: w285 -> [w302]
          frame #0 {
            n147 = property on="Y Position SP mm" class="DigNum (strict)"() -> ("Value"=w293:dbl)  [unwired: 2 in, 2 out]
            n148 = property on="Y offset mm" class="DigNum (strict)"() -> ("Value"=w294:dbl)  [unwired: 2 in, 2 out]
            n149 = Subtract(x=w293, y=w294) -> (x-y=w298:dbl)
            n150 = property on="Y mm/rev" class="DigNum (strict)"() -> ("Value"=w297:dbl)  [unwired: 2 in, 2 out]
            n151 = property on="Y steps/rev" class="DigNum (strict)"() -> ("Value"=w296:u32)  [unwired: 2 in, 2 out]
            n152 = Divide(x=w298, y=w297) -> (x/y=w299:dbl)
            n153 = To Double Precision Float(number=w296) -> (double precision float=w300:dbl)
            n154 = Multiply(x=w299, y=w300) -> (x*y=w292:dbl)
            n155 = In Range and Coerce(upper limit=w290, x=w292, lower limit=w291) -> (coerced(x)=w289:dbl)  [unwired: 1 out]
            n156 = To Long Integer(number=w289) -> (32bit integer=w295:i32)
            n157 = property on="Y Step SP" class="DigNum (strict)"("Val(Sgnl)"=w295) -> ()  [unwired: 2 in, 2 out]
          }
          frame #1 {
            n158 = property on="Y Velocity SP mm/sec" class="DigNum (strict)"() -> ("Value"=w308:dbl)  [unwired: 2 in, 2 out]
            n159 = property on="Y mm/rev" class="DigNum (strict)"() -> ("Value"=w310:dbl)  [unwired: 2 in, 2 out]
            n160 = property on="Y steps/rev" class="DigNum (strict)"() -> ("Value"=w306:u32)  [unwired: 2 in, 2 out]
            n161 = Divide(x=w308, y=w310) -> (x/y=w309:dbl)
            n162 = To Double Precision Float(number=w306) -> (double precision float=w307:dbl)
            n163 = Multiply(x=w309, y=w307) -> (x*y=w304:dbl)
            n164 = In Range and Coerce(upper limit=w303, x=w304, lower limit=w302) -> (coerced(x)=w301:dbl)  [unwired: 1 out]
            n165 = To Long Integer(number=w301) -> (32bit integer=w305:i32)
            n166 = property on="Y Velocity SP step/sec" class="DigNum (strict)"("Val(Sgnl)"=w305) -> ()  [unwired: 2 in, 2 out]
          }
        }
      }
      event #5 {
        n167 = event-data() -> ()  [unwired: 1 in, 7 out]
        n168 = flat-sequence {
          tunnel: w312 -> [w316]
          tunnel: w311 -> [w315]
          tunnel: w314 -> [w326]
          tunnel: w313 -> [w325]
          frame #0 {
            n169 = property on="Y Scan Length SP mm" class="DigNum (strict)"() -> ("Value"=w319:dbl)  [unwired: 2 in, 2 out]
            n170 = property on="Y mm/rev" class="DigNum (strict)"() -> ("Value"=w322:dbl)  [unwired: 2 in, 2 out]
            n171 = property on="Y steps/rev" class="DigNum (strict)"() -> ("Value"=w321:u32)  [unwired: 2 in, 2 out]
            n172 = Divide(x=w319, y=w322) -> (x/y=w323:dbl)
            n173 = To Double Precision Float(number=w321) -> (double precision float=w324:dbl)
            n174 = Multiply(x=w323, y=w324) -> (x*y=w318:dbl)
            n175 = In Range and Coerce(upper limit=w315, x=w318, lower limit=w316) -> (coerced(x)=w317:dbl)  [unwired: 1 out]
            n176 = To Long Integer(number=w317) -> (32bit integer=w320:i32)
            n177 = property on="Y Scan Length SP steps" class="DigNum (strict)"("Val(Sgnl)"=w320) -> ()  [unwired: 2 in, 2 out]
          }
          frame #1 {
            n178 = property on="Y Scan Velocity SP mm/sec" class="DigNum (strict)"() -> ("Value"=w332:dbl)  [unwired: 2 in, 2 out]
            n179 = property on="Y steps/rev" class="DigNum (strict)"() -> ("Value"=w330:u32)  [unwired: 2 in, 2 out]
            n180 = property on="Y mm/rev" class="DigNum (strict)"() -> ("Value"=w334:dbl)  [unwired: 2 in, 2 out]
            n181 = Divide(x=w332, y=w334) -> (x/y=w333:dbl)
            n182 = To Double Precision Float(number=w330) -> (double precision float=w331:dbl)
            n183 = Multiply(x=w333, y=w331) -> (x*y=w328:dbl)
            n184 = In Range and Coerce(upper limit=w326, x=w328, lower limit=w325) -> (coerced(x)=w327:dbl)  [unwired: 1 out]
            n185 = To Long Integer(number=w327) -> (32bit integer=w329:i32)
            n186 = property on="Y Scan Velocity SP steps/sec" class="DigNum (strict)"("Val(Sgnl)"=w329) -> ()  [unwired: 2 in, 2 out]
          }
        }
      }
      event #6 {
        n187 = event-data() -> ()  [unwired: 1 in, 7 out]
        n188 = flat-sequence {
          tunnel: w339 -> [w349]
          tunnel: w340 -> [w350]
          tunnel: [w350] -> w336
          tunnel: [w349] -> w335
          tunnel: [w353] -> w338
          tunnel: [w352] -> w337
          tunnel: w336 -> [w355]
          tunnel: w335 -> [w354]
          tunnel: [w373] -> w342
          tunnel: [w372] -> w341
          tunnel: w338 -> [w371]
          tunnel: w337 -> [w370]
          tunnel: [w380] -> w344
          tunnel: [w379] -> w343
          tunnel: w342 -> [w378]
          tunnel: w341 -> [w377]
          tunnel: [w386] -> w345
          tunnel: [w387] -> w346
          tunnel: w344 -> [w387]
          tunnel: w343 -> [w385]
          frame #0 {
            n189 = property on="Go" class="Bool"("DisabledEnum"=T1."Disabled and Grayed Out" ("Disabled")) -> ()  [unwired: 2 in, 2 out]
            n190 = property on="Scan Go" class="Bool"("DisabledEnum"=T1."Disabled and Grayed Out" ("Disabled")) -> ()  [unwired: 2 in, 2 out]
          }
          frame #1 {
            n191 = property on="Y Step SP" class="DigNum (strict)"() -> ("Value"=w363:i32)  [unwired: 2 in, 2 out]
            n192 = property on="Y Step PV" class="DigNum (strict)"() -> ("Value"=w362:i32)  [unwired: 2 in, 2 out]
            n193 = Subtract(x=w363, y=w362) -> (x-y=w361:i32)
            n194 = property on="Y Backlash" class="DigNum (strict)"() -> ("Value"=w351:i32)  [unwired: 2 in, 2 out]
            n195 = Sign(1:w351) -> (0:w359:i32)
            n196 = Sign(1:w361) -> (0:w360:i32)
            n197 = Multiply(x=w360, y=w359) -> (x*y=w358:i32)
            n198 = Equal?(x=w358, y=1) -> (x = y?=w356:bool)
            n199 = case shown="False" w356 {
              tunnel: w355 -> [w366 w368]
              tunnel: w354 -> [w365 w367]
              tunnel: [w365 w367] -> w353
              tunnel: [w366 w368] -> w352
              frame #0 {
                n200 = property on="Y Backlash corr" class="Bool (strict)"("Val(Sgnl)"=FALSE ("Value (Signaling)")) -> ()  [unwired: 2 in, 2 out]
              }
              frame #1 {
                n201 = property on="Y Backlash corr" class="Bool (strict)"("Val(Sgnl)"=TRUE ("Value (Signaling)")) -> ()  [unwired: 2 in, 2 out]
              }
            }
          }
          frame #2 {
            # "Velocity Setting"
            n202 = property on="Y Velocity SP step/sec" class="DigNum (strict)"() -> ("Value"=w374:i32)  [unwired: 2 in, 2 out]
            n203 = Number To Decimal String(number=w374) -> (decimal integer string=w375:string)  [unwired: 1 in]
            n204 = call "mDrive Send Command.vi"("error in (no error)"=w371, "Extra"=w375, "Command"=T2."Max Velocity", "VISA resource name"=w370) -> ("error out"=w372:errorcluster, "VISA resource name out"=w373:refnum<visa-resource-name>)  [unwired: 3 in, 1 out]
          }
          frame #3 {
            # "Move to Abs Position"
            n205 = property on="Y Step SP" class="DigNum (strict)"() -> ("Value"=w383:i32)  [unwired: 2 in, 2 out]
            n206 = Number To Decimal String(number=w383) -> (decimal integer string=w382:string)  [unwired: 1 in]
            n207 = call "mDrive Send Command.vi"("error in (no error)"=w377, "Extra"=w382, "Command"=T2."Move to Absolute Position", "VISA resource name"=w378) -> ("error out"=w379:errorcluster, "VISA resource name out"=w380:refnum<visa-resource-name>)  [unwired: 3 in, 1 out]
          }
          frame #4 {
            n208 = call "Time Delay"("error in (no error)"=w385, "Delay Time (s)"=0.1) -> ("error out"=w386:errorcluster)  [unwired: 9 in]
          }
        }
      }
      event #7 {
        n209 = event-data() -> ()  [unwired: 1 in, 4 out]
        n210 = event-data() -> ()  [unwired: 3 in, 1 out]
      }
      event #8 {
        n211 = event-data() -> ()  [unwired: 1 in, 7 out]
        n212 = call "mDrive Send Command.vi"("error in (no error)"=w394, "Command"=T2."Stop", "VISA resource name"=w395) -> ("error out"=w392:errorcluster, "VISA resource name out"=w393:refnum<visa-resource-name>)  [unwired: 4 in, 1 out]
      }
      event #9 {
        n213 = event-data() -> ()  [unwired: 1 in, 7 out]
        n214 = flat-sequence {
          tunnel: w401 -> [w411]
          tunnel: w400 -> [w410]
          tunnel: [w407] -> w398
          tunnel: [w405] -> w397
          tunnel: [w424] -> w399
          tunnel: [w425] -> w396
          tunnel: w398 -> [w425]
          tunnel: w397 -> [w424]
          frame #0 {
            # "VELOCITY"
            n215 = property on="Y Scan Velocity SP steps/sec" class="DigNum (strict)"() -> ("Value"=w408:i32)  [unwired: 2 in, 2 out]
            n216 = Number To Decimal String(number=w408) -> (decimal integer string=w409:string)  [unwired: 1 in]
            n217 = call "mDrive Send Command.vi"("error in (no error)"=w411, "Extra"=w409, "Command"=T2."Max Velocity", "VISA resource name"=w410) -> ("error out"=w412:errorcluster, "VISA resource name out"=w417:refnum<visa-resource-name>)  [unwired: 3 in, 1 out]
            n218 = call "Time Delay5"("error in (no error)"=w412) -> ("error out"=w415:errorcluster)  [unwired: 10 in]
            n219 = call "mDrive Send Command.vi"("error in (no error)"=w415, "Extra"="VM", "Command"=T2."Print Parameter", "VISA resource name"=w417) -> ("error out"=w406:errorcluster, "read buffer"=w413:string, "VISA resource name out"=w407:refnum<visa-resource-name>)  [unwired: 3 in]
            n220 = call "Time Delay6"("error in (no error)"=w406) -> ("error out"=w405:errorcluster)  [unwired: 10 in]
            n221 = Decimal String To Number(string=w413, offset=0) -> (number=w416:i32)  [unwired: 1 in, 1 out]
            n222 = property on="Y scan steps/sec MV step/sec" class="DigNum (strict)"("Val(Sgnl)"=w416) -> ()  [unwired: 2 in, 2 out]
          }
          frame #1 {
            n223 = property on="Y Scan" class="Bool (strict)"("Val(Sgnl)"=TRUE ("Slew Ready 2")) -> ()  [unwired: 2 in, 2 out]
            n224 = property on="Scan Go" class="Bool"("DisabledEnum"=T1."Enabled" ("Disabled")) -> ()  [unwired: 2 in, 2 out]
            n225 = property on="Y Scan Cancel" class="Bool"("DisabledEnum"=T1."Enabled" ("Disabled")) -> ()  [unwired: 2 in, 2 out]
            n226 = property on="Y Scan Length SP steps" class="DigNum (strict)"("DisabledEnum"=T1."Disabled and Grayed Out" ("Disabled")) -> ()  [unwired: 2 in, 2 out]
            n227 = property on="Go" class="Bool"("DisabledEnum"=T1."Disabled and Grayed Out" ("Disabled")) -> ()  [unwired: 2 in, 2 out]
            n228 = property on="Y Scan Velocity SP steps/sec" class="DigNum (strict)"("DisabledEnum"=T1."Disabled and Grayed Out" ("Disabled")) -> ()  [unwired: 2 in, 2 out]
          }
        }
      }
      event #10 {
        n229 = event-data() -> ()  [unwired: 1 in, 7 out]
        n230 = property on="Y Scan" class="Bool (strict)"("Value"=FALSE ("Slew Ready")) -> ()  [unwired: 2 in, 2 out]
        n231 = property on="Y Scan Length SP steps" class="DigNum (strict)"("DisabledEnum"=T1."Enabled" ("Disabled")) -> ()  [unwired: 2 in, 2 out]
        n232 = property on="Go" class="Bool"("DisabledEnum"=T1."Enabled" ("Disabled")) -> ()  [unwired: 2 in, 2 out]
        n233 = property on="Y Scan Set" class="Bool"("DisabledEnum"=T1."Enabled" ("Disabled")) -> ()  [unwired: 2 in, 2 out]
        n234 = property on="Y Scan Velocity SP steps/sec" class="DigNum (strict)"("DisabledEnum"=T1."Enabled" ("Disabled")) -> ()  [unwired: 2 in, 2 out]
        n235 = property on="Y Scan Set" class="Bool"("DisabledEnum"=T1."Enabled" ("Disabled")) -> ()  [unwired: 2 in, 2 out]
        n236 = property on="Y Scan Cancel" class="Bool"("DisabledEnum"=T1."Disabled and Grayed Out" ("Disabled")) -> ()  [unwired: 2 in, 2 out]
        n237 = property on="Scan Go" class="Bool"("DisabledEnum"=T1."Disabled and Grayed Out" ("Disabled")) -> ()  [unwired: 2 in, 2 out]
        n238 = call "mDrive Send Command.vi"("error in (no error)"=w431, "Command"=T2."Stop", "VISA resource name"=w432) -> ("error out"=w433:errorcluster, "VISA resource name out"=w434:refnum<visa-resource-name>)  [unwired: 4 in, 1 out]
        n239 = property on="Scan Go" class="Bool" props=["DisabledEnum"]() -> ()  [unwired: 2 in, 3 out]
      }
      event #11 {
        n240 = event-data() -> ()  [unwired: 1 in, 7 out]
        n241 = property on="Y Scan" class="Bool (strict)"() -> ("Value"=w442:bool)  [unwired: 2 in, 2 out]
        n242 = flat-sequence {
          tunnel: w455 -> [w458]
          tunnel: w454 -> [w459]
          tunnel: [w459] -> w451
          tunnel: [w458] -> w450
          tunnel: [w457] -> w449
          tunnel: w442 -> [w456]
          tunnel: [w456] -> w441
          tunnel: w451 -> [w470]
          tunnel: [w472] -> w446
          tunnel: w450 -> [w469]
          tunnel: [w471] -> w444
          tunnel: w449 -> [w468]
          tunnel: w441 -> [w467]
          tunnel: [w467] -> w439
          tunnel: w446 -> [w483]
          tunnel: [w483] -> w445
          tunnel: w444 -> [w482]
          tunnel: [w482] -> w443
          tunnel: [w480] -> w440
          tunnel: w439 -> [w480]
          tunnel: w445 -> [w488]
          tunnel: [w486] -> w448
          tunnel: w443 -> [w487]
          tunnel: [w485] -> w447
          tunnel: w440 -> [w484]
          tunnel: w448 -> [w503]
          tunnel: w447 -> [w502]
          tunnel: [w503] -> w453
          tunnel: [w502] -> w452
          frame #0 {
            n243 = case shown="True" w456 {
              tunnel: ["" w461] -> w457
              frame #0 {
              }
              frame #1 {
                n244 = property on="Y Scan Length SP steps" class="DigNum (strict)"() -> ("Value"=w466:i32)  [unwired: 2 in, 2 out]
                n245 = Number To Decimal String(number=w466) -> (decimal integer string=w463:string)  [unwired: 1 in]
                n246 = call <vilib>:"Space Constant.vi"() -> ("String"=w464:string)
                n247 = Concatenate Strings("MR", w464, w463, "\r") -> (w461:string)
              }
            }
          }
          frame #1 {
            n248 = case shown="True" w467 {
              tunnel: [w474 w479] -> w472
              tunnel: [w473 w478] -> w471
              tunnel: w470 -> [w474 w477]
              tunnel: w469 -> [w473 w476]
              tunnel: w468 -> [_ w475]
              frame #0 {
              }
              frame #1 {
                n249 = VISA Write(VISA resource name=w477, write buffer=w475, error in (no error)=w476) -> (VISA resource name out=w479:refnum<visa-resource-name>, error out=w478:errorcluster)  [unwired: 1 out]
              }
            }
          }
          frame #2 {
            n250 = call "Time Delay7"("Delay Time (s)"=0.1) -> ()  [unwired: 10 in, 1 out]
          }
          frame #3 {
            n251 = case shown="True" w484 {
              tunnel: w488 -> [w490 w494]
              tunnel: w487 -> [w489 w493]
              tunnel: [w490 w492] -> w486
              tunnel: [w489 w491] -> w485
              frame #0 {
              }
              frame #1 {
                n252 = property class="Instr"(reference=w494, error in=w493) -> (reference out=w496:refnum<visa-resource-name>, error out=w495:errorcluster, "Serial Settings:Number of Bytes at Serial Port"=w497:u32)
                n253 = VISA Read(VISA resource name=w496, byte count=w497, error in (no error)=w495) -> (VISA resource name out=w492:refnum<visa-resource-name>, error out=w491:errorcluster)  [unwired: 2 out]
              }
            }
          }
          frame #4 {
            n254 = property on="Y Scan" class="Bool (strict)"("Val(Sgnl)"=FALSE ("Slew Ready 2")) -> ()  [unwired: 2 in, 2 out]
            n255 = property on="Y Scan Length SP steps" class="DigNum (strict)"("DisabledEnum"=T1."Enabled" ("Disabled")) -> ()  [unwired: 2 in, 2 out]
            n256 = property on="Slew Velocity" class="DigNum (strict)"("DisabledEnum"=T1."Enabled" ("Disabled")) -> ()  [unwired: 2 in, 2 out]
            n257 = property on="Scan Go" class="Bool"("DisabledEnum"=T1."Disabled and Grayed Out" ("Disabled")) -> ()  [unwired: 2 in, 2 out]
          }
        }
      }
      event #12 {
        n258 = event-data() -> ()  [unwired: 1 in, 7 out]
        n259 = property on="Reset Y Motor Steps" class="DigNum (strict)"() -> ("Value"=w508:i32)  [unwired: 2 in, 2 out]
        n260 = Number To Decimal String(number=w508) -> (decimal integer string=w509:string)  [unwired: 1 in]
        n261 = call "mDrive Send Command.vi"("error in (no error)"=w506, "Extra"=w509, "Command"=T2."Set Current Position", "VISA resource name"=w507) -> ("error out"=w504:errorcluster, "VISA resource name out"=w505:refnum<visa-resource-name>)  [unwired: 3 in, 1 out]
      }
    }
  }
  n262 = To Long Integer(number=w27) -> (32bit integer=w33:i32)
  n263 = property on="Y Step SP" class="DigNum (strict)"("Maximum"=w28) -> ()  [unwired: 2 in, 2 out]
  n264 = property on="Y Step SP" class="DigNum (strict)"("Val(Sgnl)"=w33) -> ()  [unwired: 2 in, 2 out]
  n265 = property on="Y Step SP" class="DigNum (strict)"("Minimum"=w29) -> ()  [unwired: 2 in, 2 out]
  n266 = In Range and Coerce(upper limit=w28, x=w33, lower limit=w29) -> (In Range?=w30:bool)  [unwired: 1 out]
  n267 = property on="Y in Range" class="Bool (strict)"("Val(Sgnl)"=w30) -> ()  [unwired: 2 in, 2 out]
  n268 = flat-sequence {
    tunnel: w32 -> [w515]
    tunnel: w31 -> [w512]
    frame #0 {
      n269 = call "mDrive Send Command.vi"("error in (no error)"=w512, "Command"=T2."Stop", "VISA resource name"=w515) -> ("error out"=w513:errorcluster, "VISA resource name out"=w514:refnum<visa-resource-name>)  [unwired: 4 in, 1 out]
      n270 = VISA Close(VISA resource name=w514, error in (no error)=w513) -> ()  [unwired: 1 out]
    }
  }
  "Y COM PORT" <- w36
  "Y MINPOS" <- w29
  "Y MAXPOS" <- w28
  "Y steps/rev" <- w6
  "Y mm/rev" <- w9
  "Y offset mm" <- 0.0 ("offset")
  "Y Run Current %" <- 60 ("Run Current %")
  "Y Holding Current %" <- 25 ("Holding Current %")
  "Y Backlash" <- -5120 ("Backlash2")
  "Y Backlash steps/sec" <- 25600 ("Value (Signaling)")
